vi "RT_TVA_DATA_v2.vi"(11 "TVA_Data":u64[](array[numeric])) -> (0 "Yaw stream":dbl, 1 "Roll DMARS":dbl, 2 "Yaw Angle":dbl(knob) scale=-3.0..3.0, 3 "Pitch Angle":dbl(knob) scale=-3.0..3.0, 4 "Data CRC Fault":bool, 5 "Yaw DMARS":dbl, 6 "Address CRC Fault":bool, 7 "Pitch DMARS":dbl)   [LabVIEW 2011]
panel:
  out "DMARS Euler Angles [deg/s]":dbl[](array[numeric])
  out "Roll Angle":dbl
  out "Roll Rate":dbl
  out "element":u64 format="%x"
  out "element 4":u64 format="%x"
  out "element 3":u64 format="%x"
  out "element 2":u64 format="%x"
  out "Dest address":u8
  out "Souce address":u8
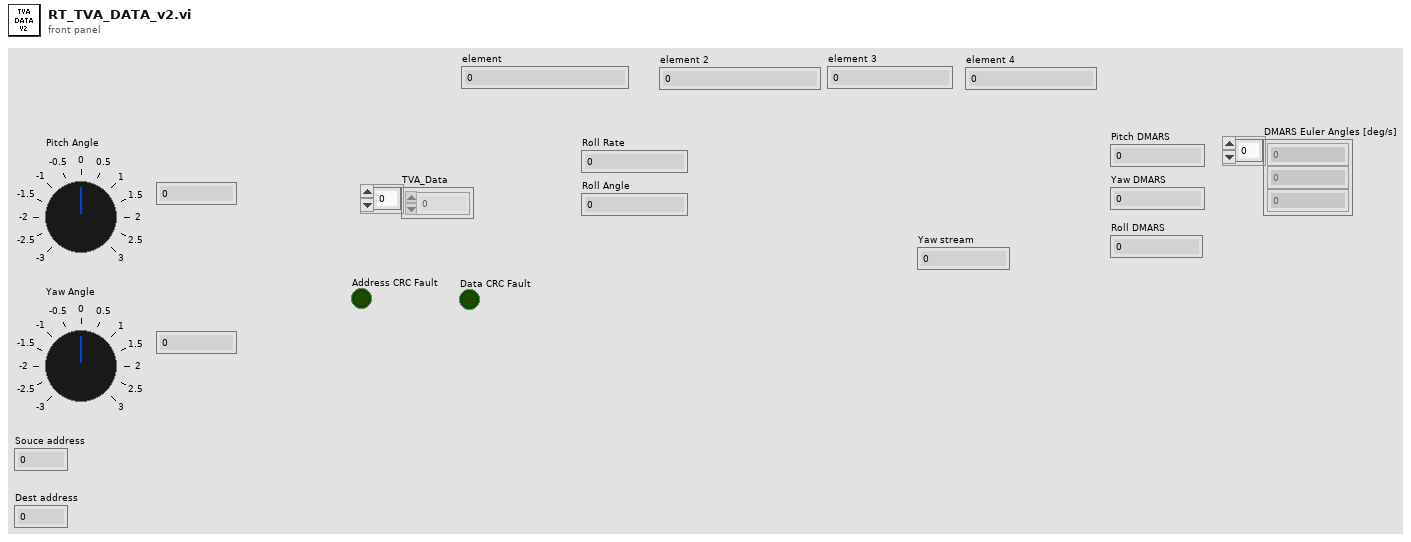
[diagram p1: front panel]
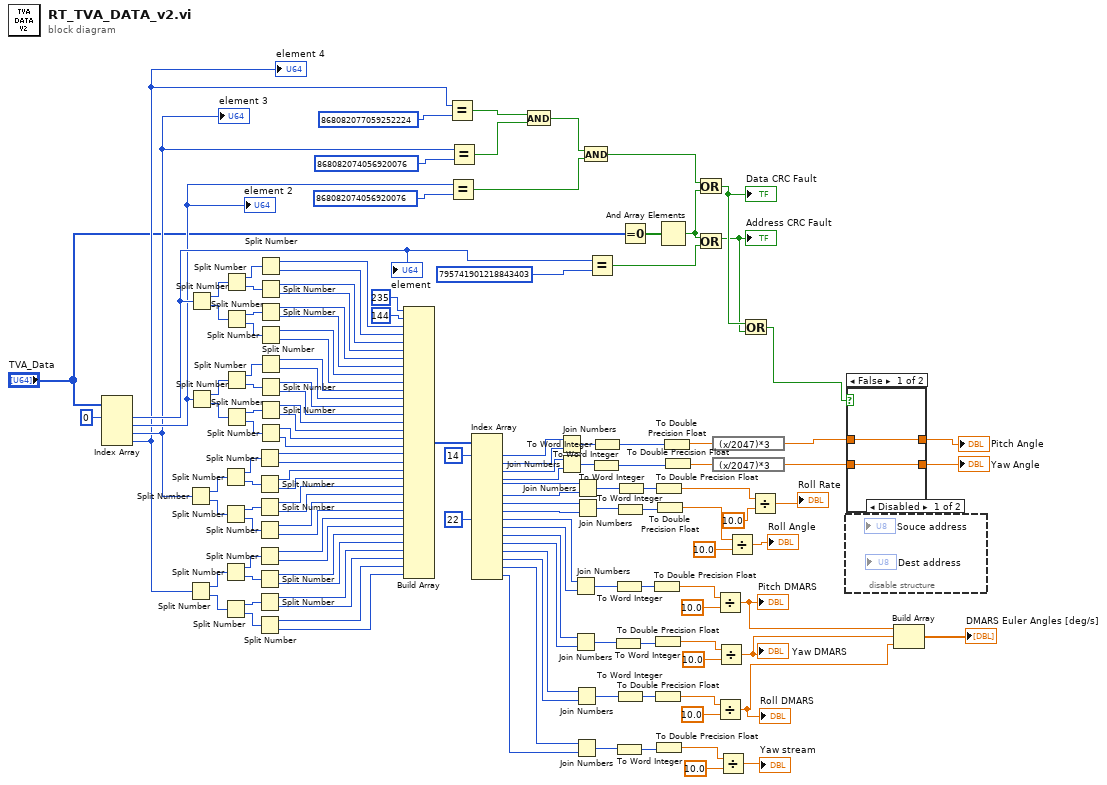
[diagram p0: block diagram]
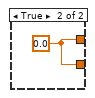
[diagram p3: hidden frame]
diagram:
  n1 = Index Array(array="TVA_Data", index #1=0 ("index")) -> (element #1=w71:u64, element #2=w68:u64, element #3=w66:u64, element #4=w64:u64)  [unwired: 3 in]
  "element 2" <- w68
  "element 3" <- w66
  "element 4" <- w64
  "element" <- w71
  n2 = Split Number(x=w66) -> (hi(x)=w87:u32, lo(x)=w88:u32)
  n3 = Split Number(x=w64) -> (hi(x)=w98:u32, lo(x)=w97:u32)
  n4 = Split Number(x=w71) -> (hi(x)=w75:u32, lo(x)=w76:u32)
  n5 = Split Number(x=w68) -> (hi(x)=w86:u32, lo(x)=w85:u32)
  n6 = Split Number(x=w87) -> (hi(x)=w89:u16, lo(x)=w90:u16)
  n7 = Split Number(x=w88) -> (hi(x)=w91:u16, lo(x)=w92:u16)
  n8 = Split Number(x=w98) -> (hi(x)=w96:u16, lo(x)=w95:u16)
  n9 = Split Number(x=w97) -> (hi(x)=w94:u16, lo(x)=w93:u16)
  n10 = Split Number(x=w75) -> (hi(x)=w77:u16, lo(x)=w78:u16)
  n11 = Split Number(x=w76) -> (hi(x)=w79:u16, lo(x)=w80:u16)
  n12 = Split Number(x=w86) -> (hi(x)=w84:u16, lo(x)=w83:u16)
  n13 = Split Number(x=w85) -> (hi(x)=w82:u16, lo(x)=w81:u16)
  n14 = Split Number(x=w89) -> (hi(x)=w114:u8, lo(x)=w115:u8)
  n15 = Split Number(x=w90) -> (hi(x)=w116:u8, lo(x)=w117:u8)
  n16 = Split Number(x=w91) -> (hi(x)=w118:u8, lo(x)=w119:u8)
  n17 = Split Number(x=w92) -> (hi(x)=w120:u8, lo(x)=w121:u8)
  n18 = Split Number(x=w96) -> (hi(x)=w122:u8, lo(x)=w123:u8)
  n19 = Split Number(x=w95) -> (hi(x)=w124:u8, lo(x)=w125:u8)
  n20 = Split Number(x=w94) -> (hi(x)=w126:u8, lo(x)=w127:u8)
  n21 = Split Number(x=w93) -> (hi(x)=w138:u8, lo(x)=w139:u8)
  n22 = Split Number(x=w77) -> (hi(x)=w99:u8, lo(x)=w100:u8)
  n23 = Split Number(x=w78) -> (hi(x)=w101:u8, lo(x)=w102:u8)
  n24 = Split Number(x=w79) -> (hi(x)=w103:u8, lo(x)=w104:u8)
  n25 = Split Number(x=w80) -> (hi(x)=w105:u8, lo(x)=w106:u8)
  n26 = Split Number(x=w84) -> (hi(x)=w72:u8, lo(x)=w107:u8)
  n27 = Split Number(x=w83) -> (hi(x)=w108:u8, lo(x)=w109:u8)
  n28 = Split Number(x=w82) -> (hi(x)=w110:u8, lo(x)=w111:u8)
  n29 = Split Number(x=w81) -> (hi(x)=w112:u8, lo(x)=w113:u8)
  n30 = Build Array(u8 235 ("x"), u8 144 ("x"), w99, w100, w101, w102, w103, w104, w105, w106, w72, w107, w108, w109, w110, w111, w112, w113, w114, w115, w116, w117, w118, w119, w120, w121, w122, w123, w124, w125, w126, w127, w138, w139) -> (w128:u8[])
  n31 = Equal?(x=w64, y=u64 868082077059252224) -> (x = y?=w63:bool)
  n32 = Equal?(x=w68, y=u64 868082074056920076) -> (x = y?=w60:bool)
  n33 = Equal?(x=w66, y=u64 868082074056920076) -> (x = y?=w62:bool)
  n34 = Index Array(array=w128, index #1=14 ("index"), index #9=22 ("index")) -> (element #1=w132:u8, element #2=w133:u8, element #3=w134:u8, element #4=w135:u8, element #5=w48:u8, element #6=w47:u8, element #7=w46:u8, element #8=w45:u8, element #9=w7:u8, element #10=w8:u8, element #11=w6:u8, element #12=w5:u8, element #13=w21:u8, element #14=w20:u8, element #15=w19:u8, element #16=w18:u8)  [unwired: 14 in]
  n35 = And(x=w63, y=w62) -> (x .and. y?=w61:bool)
  n36 = Join Numbers(hi=w132, lo=w133) -> ((hi.lo)=w38:u16)
  n37 = Join Numbers(hi=w134, lo=w135) -> ((hi.lo)=w36:u16)
  n38 = Join Numbers(hi=w7, lo=w8) -> ((hi.lo)=w26:u16)
  n39 = Join Numbers(hi=w6, lo=w5) -> ((hi.lo)=w27:u16)
  n40 = Join Numbers(hi=w21, lo=w20) -> ((hi.lo)=w25:u16)
  n41 = Join Numbers(hi=w19, lo=w18) -> ((hi.lo)=w24:u16)
  n42 = Join Numbers(hi=w48, lo=w47) -> ((hi.lo)=w34:u16)
  n43 = Join Numbers(hi=w46, lo=w45) -> ((hi.lo)=w33:u16)
  n44 = And(x=w61, y=w60) -> (x .and. y?=w56:bool)
  n45 = Equal?(x=w71, y=u64 795741901218843403) -> (x = y?=w70:bool)
  n46 = To Word Integer(number=w36) -> (16bit integer=w35:i16)
  n47 = To Word Integer(number=w38) -> (16bit integer=w37:i16)
  n48 = To Word Integer(number=w27) -> (16bit integer=w28:i16)
  n49 = To Word Integer(number=w26) -> (16bit integer=w29:i16)
  n50 = To Word Integer(number=w24) -> (16bit integer=w23:i16)
  n51 = To Word Integer(number=w33) -> (16bit integer=w32:i16)
  n52 = To Word Integer(number=w25) -> (16bit integer=w22:i16)
  n53 = To Word Integer(number=w34) -> (16bit integer=w31:i16)
  n54 = Equal To 0?(x="TVA_Data") -> (x = 0?=w58:bool[])
  n55 = To Double Precision Float(number=w29) -> (double precision float=w16:dbl)
  n56 = To Double Precision Float(number=w28) -> (double precision float=w12:dbl)
  n57 = To Double Precision Float(number=w22) -> (double precision float=w11:dbl)
  n58 = To Double Precision Float(number=w31) -> (double precision float=w39:dbl)
  n59 = To Double Precision Float(number=w23) -> (double precision float=w10:dbl)
  n60 = To Double Precision Float(number=w32) -> (double precision float=w41:dbl)
  n61 = And Array Elements(Boolean array=w58) -> (logical AND=w57:bool)
  n62 = To Double Precision Float(number=w37) -> (double precision float=w137:dbl)
  n63 = To Double Precision Float(number=w35) -> (double precision float=w136:dbl)
  n64 = Or(x=w56, y=w57) -> (x .or. y?=w55:bool)
  "Data CRC Fault" <- w55
  n65 = Or(x=w57, y=w70) -> (x .or. y?=w54:bool)
  "Address CRC Fault" <- w54
  n66 = expression code="(x/2047)*3"(w137) -> (w50:dbl)
  n67 = expression code="(x/2047)*3"(w136) -> (w49:dbl)
  n68 = Divide(x=w16, y=10.0) -> (x/y=w4:dbl)
  "Pitch DMARS" <- w4
  n69 = Divide(x=w11, y=10.0) -> (x/y=w2:dbl)
  "Roll DMARS" <- w2
  n70 = Divide(x=w12, y=10.0) -> (x/y=w3:dbl)
  "Yaw DMARS" <- w3
  n71 = Divide(x=w10, y=10.0) -> (x/y=→"Yaw stream":dbl)
  n72 = Divide(x=w41, y=10.0) -> (x/y=→"Roll Angle":dbl)
  n73 = Or(x=w55, y=w54) -> (x .or. y?=w53:bool)
  n74 = Divide(x=w39, y=10.0) -> (x/y=→"Roll Rate":dbl)
  n75 = disable-structure shown="Disabled" {
    frame Disabled {
    }
    frame Enabled {
    }
  }
  n76 = case shown="False" w53 {
    tunnel: [w141 w142] -> w52
    tunnel: [w140 w142] -> w51
    tunnel: w50 -> [w141 _]
    tunnel: w49 -> [w140 _]
    frame False {
    }
    frame True {
      w142 = 0.0
    }
  }
  "Yaw Angle" <- w51
  "Pitch Angle" <- w52
  n77 = Build Array(w4, w3, w2) -> (→"DMARS Euler Angles [deg/s]":dbl[])
